vi "Transmit and Receive Messages with Explicit Schedule.vi"() -> ()   [LabVIEW 2019]
doc: "This example opens the specified card and core. The provided XML Configuration\nbuilds a transmit schedule using explicit message timing, configures a receive\nchannel and enables the self-test wraparound. The minimum and maximum\nelasped time for each message is displayed."
uses:
  <instrlib>/BTI429Lib/Public/Controls/429 Message Fields.ctl
  <instrlib>/BTICardLib/Private/Initialize By Card Number and Core Number.vi
  <instrlib>/BTICardLib/Private/Configure Core From XML.vi
  <instrlib>/BTI429Lib/Private/Tx/Configure/Configure Tx Channel From XML.vi
  <instrlib>/BTI429Lib/Private/Rx/Configure/Configure Rx Channel From XML.vi
  <instrlib>/BTI429Lib/Private/Rx/Configure/Get Rx Label Handle Name.vi
  <instrlib>/BTI429Lib/Private/Core/Action-Status/Start All Channels.vi
  <instrlib>/BTI429Lib/Private/Core/Action-Status/Stop All Channels.vi
  <instrlib>/BTICardLib/BTICardLV.lvlib
  <instrlib>/BTI429Lib/BTI429LV.lvlib
panel:
  out "core number":i32
  out "tx channel number":i32
  out "rx channel number":i32
  in  "Rx Channel XML Configuration File Name":string="Channel Config Rx.xml"
  out "Airspeed":T1 {"speed" items=["CHSPEED429_LOW", "CHSPEED429_HIGH"]; "msgdata" format="%08x"; "timetagh" format="%08x"; "timetag_hitcount" format="%08x"; "maxtime_elapsetime" format="%08x"; "mintime" format="%08x"; "paramflag" format="%04x"}
  out "Altitude":T1 {"speed" items=["CHSPEED429_LOW", "CHSPEED429_HIGH"]; "msgdata" format="%08x"; "timetagh" format="%08x"; "timetag_hitcount" format="%08x"; "maxtime_elapsetime" format="%08x"; "mintime" format="%08x"; "paramflag" format="%04x"}
  in  "Tx Channel XML Configuration File Name":string="Channel Config Tx.xml"
  in  "Core XML Configuration File Name":string="Core Config.xml"
  in  "Card Number":i32
  in  "stop":bool
  out "error out":errorcluster
  # "ARINC 429: Transmit and Receive with Explicit Schedule"
  # "©2016 Astronics Ballard Technology"
  # "This example opens the specified card and core. The provided XML Configuration\nbuilds a transmit schedule using explicit message timing, configures a receive\nchannel and enables the self-test wraparound. The minimum and maximum\nelasped time for each message is displayed."
  # "Always Stop the card\nand Close the card when\ndone. Otherwise, the hardware\ncontinues to operate."
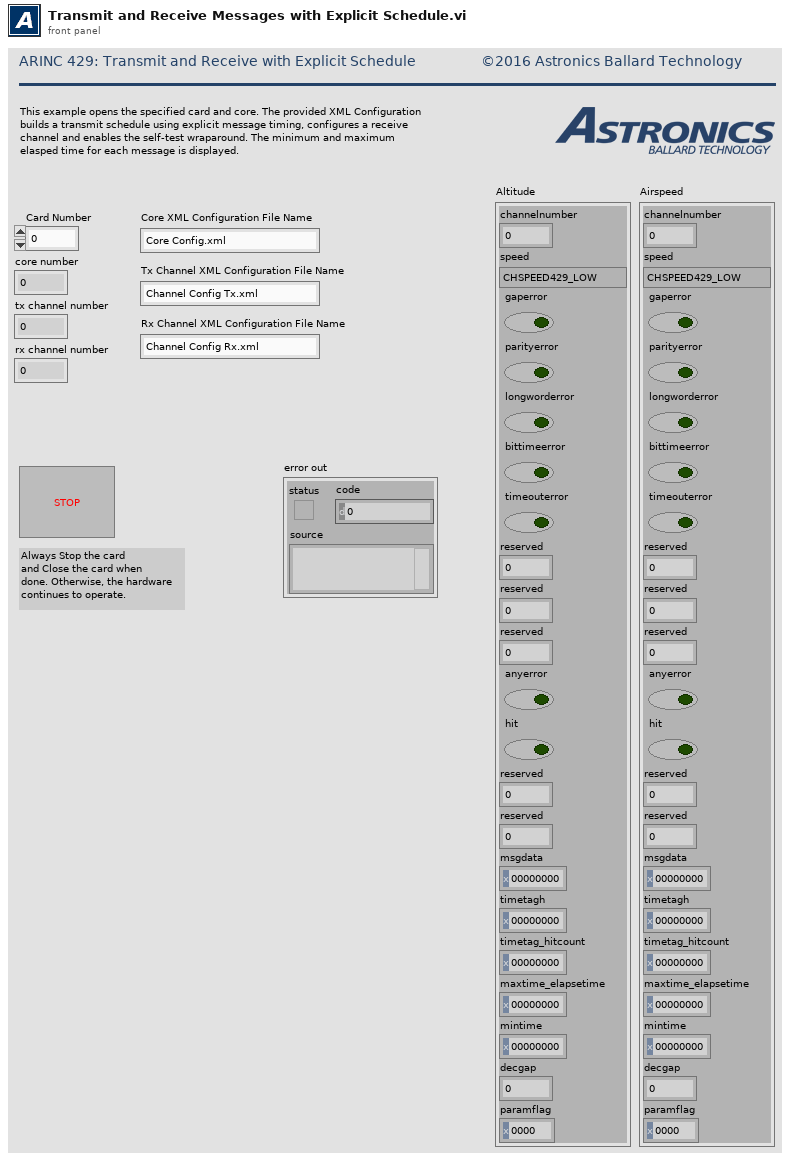
[diagram p1: front panel]
types:
  T1 = typedef "BTI429LV.lvlib/429 Message Fields.ctl" = cluster{"channelnumber":i32, "speed":u32, "gaperror":bool, "parityerror":bool, "longworderror":bool, "bittimeerror":bool, "timeouterror":bool, "reserved":i8, "reserved":i8, "reserved":i8, "anyerror":bool, "hit":bool, "reserved":i8, "reserved":i8, "msgdata":u32, "timetagh":u32, "timetag_hitcount":u32, "maxtime_elapsetime":u32, "mintime":u32, "decgap":u16, "paramflag":u16}
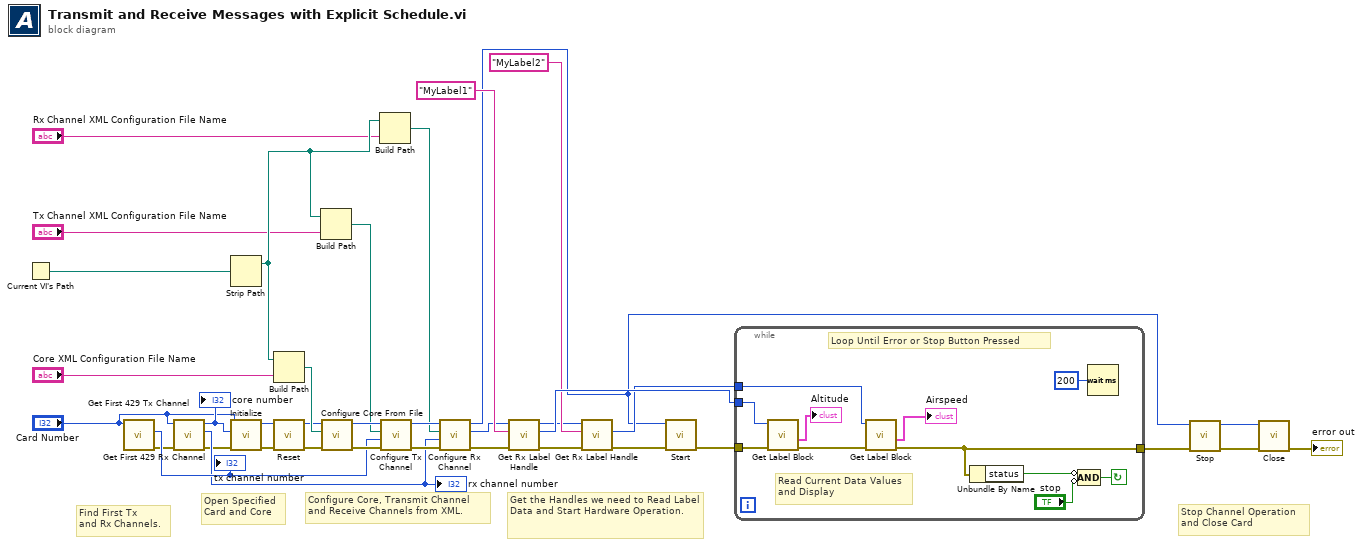
[diagram p0: block diagram]
diagram:
  # "Find First Tx \nand Rx Channels."
  # "Stop Channel Operation\nand Close Card"
  # "Get the Handles we need to Read Label Data and Start Hardware Operation."
  # "Configure Core, Transmit Channel\nand Receive Channels from XML."
  # "Open Specified\nCard and Core"
  n1 = Current VI's Path() -> (path=w25:path)
  n2 = call "Get First 429 Tx Channel.vi"("Card Number"="Card Number") -> ("error out"=w2:errorcluster, "Channel Number"=w4:i32)  [unwired: 8 in, 1 out]
  "tx channel number" <- w4
  n3 = call "Get First 429 Rx Channel.vi"("error in (no error)"=w2, "Card Number"="Card Number") -> ("error out"=w1:errorcluster, "Channel Number"=w3:i32, "Core Number"=w6:i32)  [unwired: 7 in]
  "rx channel number" <- w3
  "core number" <- w6
  n4 = Strip Path(path=w25) -> (stripped path=w16:path)  [unwired: 1 out]
  n5 = call-poly <instrlib>:"Initialize.vi"("error in (no error)"=w1, "core number"=w6, "card number"="Card Number") -> ("error out"=w8:errorcluster, "core handle out"=w7:u64)  [unwired: 7 in]
  n6 = Build Path(base path=w16, name or relative path="Core XML Configuration File Name") -> (appended path=w17:path)
  n7 = call <instrlib>:"Reset.vi"("error in (no error)"=w8, "core handle in"=w7) -> ("error out"=w9:errorcluster, "core handle out"=w10:u64)  [unwired: 8 in]
  n8 = Build Path(base path=w16, name or relative path="Tx Channel XML Configuration File Name") -> (appended path=w12:path)
  n9 = call-poly <instrlib>:"Configure Core From File.vi"("error in (no error)"=w9, "configuration file path"=w17, "core handle in"=w10) -> ("error out"=w37:errorcluster, "core handle out"=w13:u64)  [unwired: 7 in]
  n10 = Build Path(base path=w16, name or relative path="Rx Channel XML Configuration File Name") -> (appended path=w14:path)
  n11 = call-poly <instrlib>:"Configure Tx Channel.vi"("error in (no error)"=w37, "channel number in"=w4, "configuration file path"=w12, "core handle in"=w13) -> ("error out"=w21:errorcluster, "core handle out"=w22:u64)  [unwired: 5 in, 1 out]
  n12 = call-poly <instrlib>:"Configure Rx Channel.vi"("error in (no error)"=w21, "channel number in"=w3, "configuration file path"=w14, "core handle in"=w22) -> ("error out"=w20:errorcluster, "channel handle out"=w18:u64, "core handle out"=w19:u64)  [unwired: 5 in]
  n13 = call-poly <instrlib>:"Get Rx Label Handle.vi"("error in (no error)"=w20, "label name"="MyLabel1", "channel handle in"=w18) -> ("error out"=w31:errorcluster, "label handle out"=w32:u64, "channel handle out"=w23:u64)  [unwired: 6 in]
  n14 = call-poly <instrlib>:"Get Rx Label Handle.vi"("error in (no error)"=w31, "label name"="MyLabel2", "channel handle in"=w23) -> ("error out"=w30:errorcluster, "label handle out"=w28:u64)  [unwired: 6 in, 1 out]
  n15 = call-poly <instrlib>:"Start.vi"("error in (no error)"=w30, "core handle in"=w19) -> ("error out"=w29:errorcluster)  [unwired: 8 in, 1 out]
  n16 = while {
    tunnel: [w46] -> w33
    tunnel: w32 -> [w43]
    tunnel: w29 -> [w42]
    tunnel: w28 -> [w41]
    stop <- w47 continue-if-true
    # "Read Current Data Values\nand Display"
    # "Loop Until Error or Stop Button Pressed"
    n17 = call <instrlib>:"Get Label Block.vi"("error in (no error)"=w42, "label handle in"=w43) -> ("error out"=w44:errorcluster, "value"=→"Altitude":T1)  [unwired: 6 in, 2 out]
    n18 = call <instrlib>:"Get Label Block.vi"("error in (no error)"=w44, "label handle in"=w41) -> ("error out"=w46:errorcluster, "value"=→"Airspeed":T1)  [unwired: 6 in, 2 out]
    n19 = Unbundle By Name(w46) -> ("status"=w45:bool)
    n20 = Compound Arithmetic op=AND(invert w45, invert "stop") -> (w47:bool)
    n21 = Wait (ms)(milliseconds to wait=u32 200) -> ()  [unwired: 1 out]
  }
  n22 = call-poly <instrlib>:"Stop.vi"("error in (no error)"=w33, "core handle in"=w19) -> ("error out"=w36:errorcluster, "core handle out"=w34:u64)  [unwired: 8 in]
  n23 = call <instrlib>:"Close.vi"("error in (no error)"=w36, "core handle in"=w34) -> ("error out"=→"error out":errorcluster)  [unwired: 8 in, 1 out]
